vi "Read Group name.vi"(8 "error in (no error)":errorcluster, 11 "Channel Scanner Driver in":refnum<class "Channel Scanner Driver.lvclass">) -> (0 "error out":errorcluster, 2 "Group name":string="p", 3 "Channel Scanner Driver out":refnum<class "Channel Scanner Driver.lvclass">)   [LabVIEW 2019, in "Channel Scanner Driver.lvclass"]
uses:
  Channel Scanner Driver.lvclass
  Channel Scanner Driver.lvclass/Channel Scanner Driver.ctl
  Read Scan Channels.vi
  Read Next channel idx.vi
  Simple VISA Reader/Simple VISA Reader Driver.lvclass
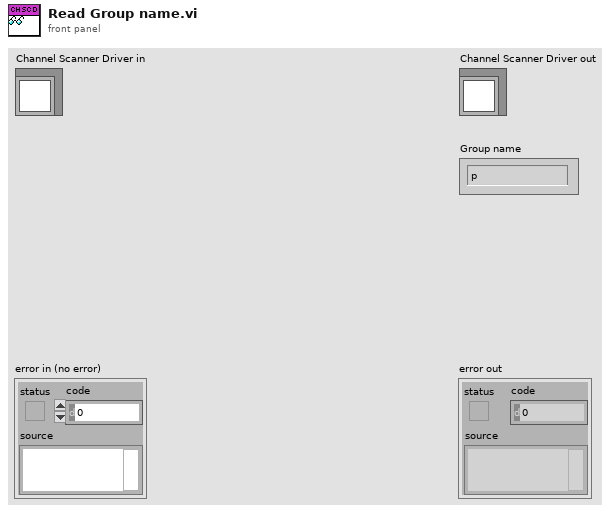
[diagram p1: front panel]
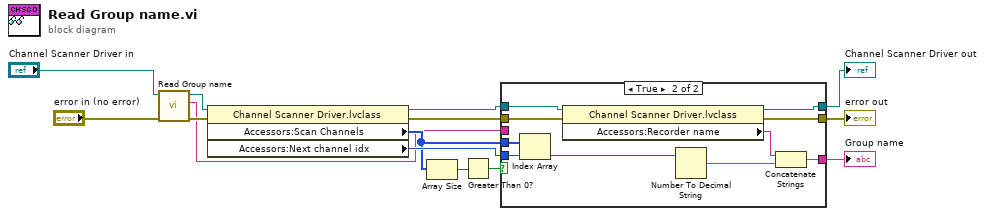
[diagram p0: block diagram]
diagram:
  n1 = call-parent "Read Group name.vi"("error in (no error)"="error in (no error)", "Instrument Driver in"="Channel Scanner Driver in") -> ("error out"=w7:errorcluster, "Group name"=w6:string, "Instrument Driver out"=w8:refnum<class "Channel Scanner Driver.lvclass">)  [unwired: 7 in]
  n2 = property class="Channel Scanner Driver.lvclass"(reference=w8, error in=w7) -> (reference out=w4:refnum<class "Channel Scanner Driver.lvclass">, error out=w3:errorcluster, "Accessors:Scan Channels"=w10:i32[], "Accessors:Next channel idx"=w11:i32)
  n3 = Array Size(array=w10) -> (size(s)=w9:i32)
  n4 = Greater Than 0?(x=w9) -> (x > 0?=w12:bool)
  n5 = case shown="True" w12 {
    tunnel: w10 -> [_ w27]
    tunnel: w11 -> [_ w26]
    tunnel: w6 -> [w17 _]
    tunnel: [w17 w23] -> w5
    tunnel: w4 -> [w16 w22]
    tunnel: w3 -> [w15 w20]
    tunnel: [w15 w19] -> w2
    tunnel: [w16 w18] -> w1
    frame False {
    }
    frame True {
      n6 = Index Array(array=w27, index=w26) -> (element=w25:i32)
      n7 = property class="Channel Scanner Driver.lvclass"(reference=w22, error in=w20) -> (reference out=w18:refnum<class "Channel Scanner Driver.lvclass">, error out=w19:errorcluster, "Accessors:Recorder name"=w21:string)
      n8 = Number To Decimal String(number=w25) -> (decimal integer string=w24:string)  [unwired: 1 in]
      n9 = Concatenate Strings(w21, w24) -> (w23:string)
    }
  }
  "error out" <- w2
  "Channel Scanner Driver out" <- w1
  "Group name" <- w5
